vi "Dpc Start Notify.vi"(8 "error in (no error)":errorcluster, 9 "perc":i32, 10 "idNotifyTemp":u16, 11 "hwndTemp":u32) -> (0 "error out":errorcluster, 1 "perc out":i32, 2 "function return":i32, 3 "hwndTemp out":u32)   [LabVIEW 2011, in "LVH-Adept.lvlib" / "DPCUTIL.lvlib"]
doc: "DPCAPI BOOL DpcStartNotify(HWND hwndTemp, WORD idNotifyTemp, ERC *perc);"
uses:
  DPCUTIL.lvlib
  dpcutil.dll
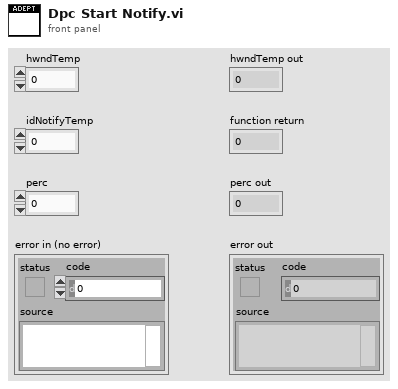
[diagram p1: front panel]
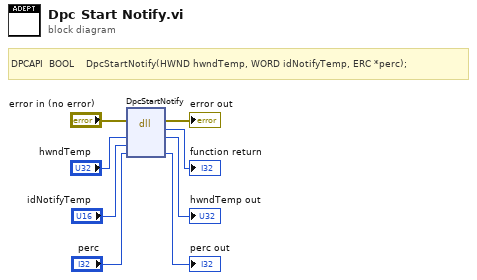
[diagram p0: block diagram]
diagram:
  # "DPCAPI  BOOL    DpcStartNotify(HWND hwndTemp, WORD idNotifyTemp, ERC *perc);"
  n1 = dll-call lib="dpcutil.*" fn="DpcStartNotify"(error in="error in (no error)", "hwndTemp"="hwndTemp", "idNotifyTemp"="idNotifyTemp", "perc"="perc") -> (error out=→"error out":errorcluster, →"function return":i32, "hwndTemp"=→"hwndTemp out":u32, "perc"=→"perc out":i32)  [unwired: 3 in, 1 out]
